vi "DAQmxTaskContainerMoveCrystal-Com-Exec.vi"(8 "error in (no error)":errorcluster, 9 "data":variant, 10 "ControlQueue":refnum<queue>, 11 "DAQmxTaksContainer_General in":refnum<class "DAQmxTaksContainer_General.lvclass">) -> (0 "error out":errorcluster, 3 "DAQmxTaksContainer_General out":refnum<class "DAQmxTaksContainer_General.lvclass">)   [LabVIEW 2020, in "DAQmxTaksContainer_General.lvclass"]
uses:
  DAQmxTaksContainer_General.lvclass
  dependecies/ControlsVIs/Clusters-def/SERVER-Commands.ctl
  dependecies/ControlsVIs/Clusters-def/ProtypeCommand-DAQmxReply.ctl
  DAQmxTask.lvclass
  Control/Control-Server/Control-Server.lvclass
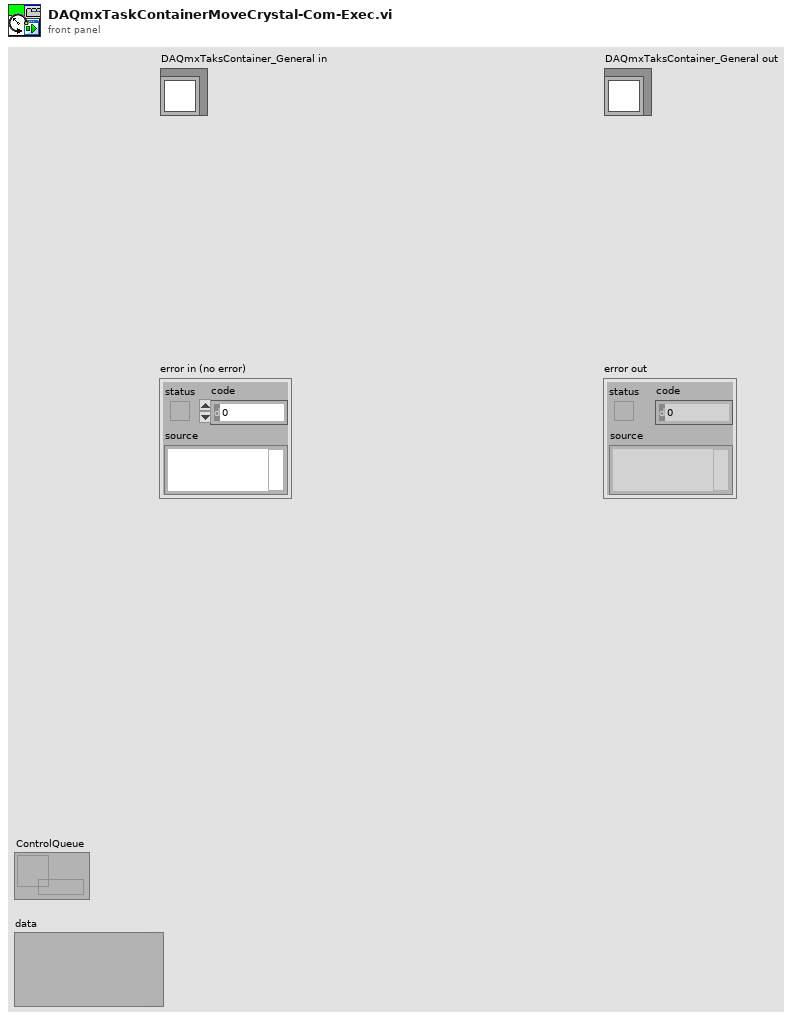
[diagram p1: front panel]
types:
  T1 = typedef "ProtypeCommand-DAQmxReply.ctl" = cluster{"On/Off":bool, "error out":errorcluster}
  T2 = typedef "Control-Server.lvclass/SERVER-Commands.ctl" = string
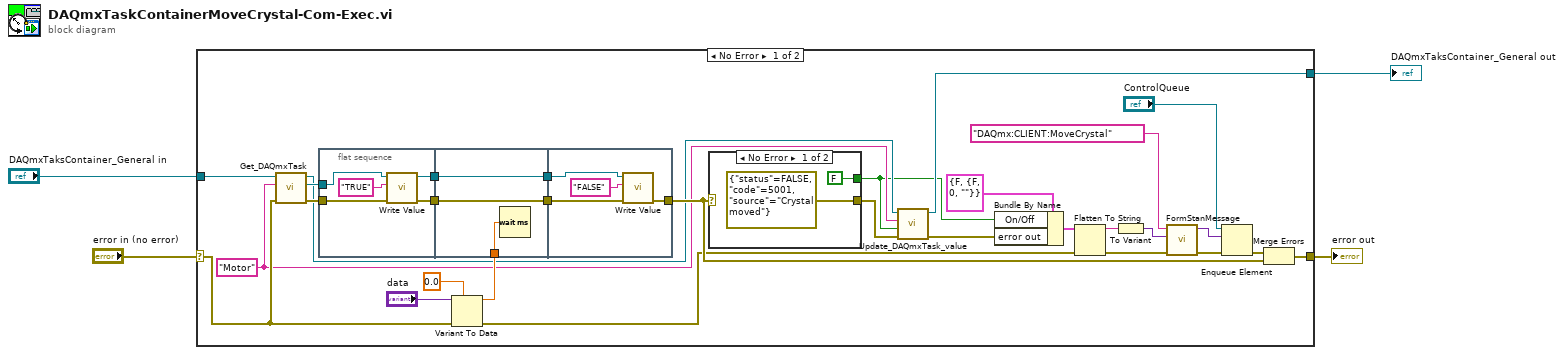
[diagram p0: block diagram]
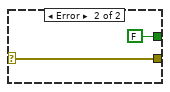
[diagram p2: hidden frame]
diagram:
  n1 = case shown="No Error" "error in (no error)" {
    selector: "error in (no error)" -> [w30 w52]
    tunnel: [w7 w51] -> w1
    tunnel: [w32 w52] -> w2
    tunnel: "DAQmxTaksContainer_General in" -> [w33 w51]
    frame No Error {
      w6 = "Motor" ("Task name")
      n2 = call "Get_DAQmxTask.vi"("error in (no error)"=w30, "Task name"=w6, "DAQmxTaksContainer_General in"=w33) -> ("error out"=w25:errorcluster, "DAQmx Task"=w23:refnum<class "DAQmxTask.lvclass">, "DAQmxTaksContainer_General out"=w10:refnum<class "DAQmxTaksContainer_General.lvclass">)  [unwired: 6 in]
      n3 = flat-sequence {
        tunnel: w25 -> [w43]
        tunnel: w23 -> [w41]
        tunnel: [w40] -> w29
        tunnel: [w39] -> w28
        tunnel: [w46] -> w27
        tunnel: w29 -> [w46]
        tunnel: w22 -> [w45]
        tunnel: [w44] -> w26
        tunnel: w28 -> [w44]
        tunnel: w27 -> [w50]
        tunnel: w26 -> [w49]
        tunnel: [w48] -> w21
        frame #0 {
          n4 = call-dynamic "Write Value.vi"("error in (no error)"=w43, "Data"="TRUE", "DAQmxTask en entrée"=w41) -> ("error out"=w39:errorcluster, "DAQmxTask en sortie"=w40:refnum<class "DAQmxTask.lvclass">)  [unwired: 7 in]
        }
        frame #1 {
          n5 = Wait (ms)(milliseconds to wait=w45) -> ()  [unwired: 1 out]
        }
        frame #2 {
          n6 = call-dynamic "Write Value.vi"("error in (no error)"=w49, "Data"="FALSE", "DAQmxTask en entrée"=w50) -> ("error out"=w48:errorcluster)  [unwired: 7 in, 1 out]
        }
      }
      n7 = Variant To Data(error in=w30, type=0.0, Variant="data") -> (data=w22:dbl, error out=w17:errorcluster)
      n8 = case shown="No Error" w21 {
        selector: w21 -> [_ w38]
        tunnel: [errorcluster {"status"=FALSE, "code"=5001, "source"="Crystal moved"} ("error constant") w38] -> w9
        tunnel: [FALSE FALSE] -> w5
        frame No Error {
        }
        frame Error {
        }
      }
      n9 = call "Update_DAQmxTask_value.vi"("error in (no error)"=w9, "Value"=w5, "Task name"=w6, "DAQmxTaksContainer_General in"=w10) -> ("error out"=w8:errorcluster, "DAQmxTaksContainer_General out"=w7:refnum<class "DAQmxTaksContainer_General.lvclass">)  [unwired: 6 in]
      n10 = Bundle By Name(cluster=T1 {"On/Off"=FALSE, "error out"={"status"=FALSE, "code"=0, "source"=""}} ("output cluster"), "On/Off"=w5, "error out"=w8) -> (w19:T1)
      n11 = Flatten To String(anything=w19, error in (no error)=w17) -> (data string=w18:string, error out=w12:errorcluster)  [unwired: 2 in, 1 out]
      n12 = To Variant(anything=w18) -> (Variant=w14:variant)
      n13 = call "FormStanMessage.vi"("error in"=w12, "data"=w14, "Command"=T2 "DAQmx:CLIENT:MoveCrystal" ("command")) -> ("error out"=w11:errorcluster, "message"=w13:variant)  [unwired: 7 in]
      n14 = Enqueue Element(queue="ControlQueue", element=w13, error in (no error)=w11) -> (error out=w16:errorcluster)  [unwired: 1 in, 2 out]
      n15 = Merge Errors(w16, w21) -> (w32:errorcluster)
    }
    frame Error {
    }
  }
  "error out" <- w2
  "DAQmxTaksContainer_General out" <- w1
